vi "setLogMode.vi"(8 "error in (no error)":errorcluster, 10 "LogMode":T1=enum."Logging", 11 "Instrument.Lockin in":refnum<class "Instrument.Lockin.lvclass">) -> (0 "error out":errorcluster, 3 "Instrument.Lockin out":refnum<class "Instrument.Lockin.lvclass">)   [LabVIEW 2019, in "Instrument.Lockin.lvlib" / "Instrument.Lockin.lvclass"]
doc: "Set the state {start, stop, reset, start sweep, stop sweep}"
uses:
  Instrument.Lockin.lvclass
  Typedefs/LogMode--Enum.ctl
  Typedefs/API/Lockin.Commands--Enum.ctl
  Typedefs/API/Lockin.setLogMode--cluster.ctl
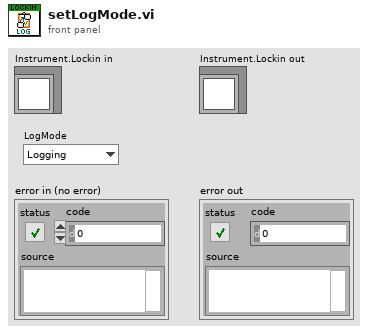
[diagram p1: front panel]
types:
  T1 = typedef "Instrument.Lockin.lvlib/Instrument.Lockin.lvclass/LogMode--Enum.ctl" = enum16{"Heartbeat", "Logging"}
  T2 = typedef "Instrument.Lockin.lvlib/Instrument.Lockin.lvclass/Lockin.setLogMode--cluster.ctl" = cluster{"LogMode":T1}
  T3 = typedef "Instrument.Lockin.lvlib/Instrument.Lockin.lvclass/Lockin.Commands--Enum.ctl" = enum16{"setAO", "setAO_Amplitude", "setAO_DC", "setAO_Frequency", "setAO_Phase", "setAO_Function", "setREF", "setREF_Frequency", "setREF_Phase", "setREF_TC", "setREF_Roll-Off", "setDAQ", "setSampling", "setState", "getState", "getAO", "getAI", "getResults", "getSampling", "getAOconfig", "getREFconfig", "setInputGain", "setOutputGain", "getInputGain", "getOutputGain", "setSamplingFsMode", "getSamplingFsMode", "setSweep", "setSweep_Time", "setSweep_Table", "getStatus", "getSweepResults", "getSweepWaveforms", "setLogMode"}
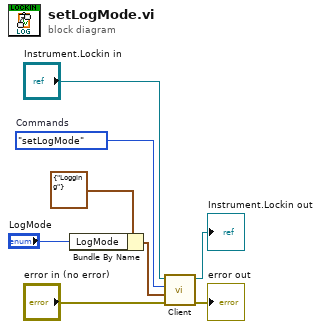
[diagram p0: block diagram]
diagram:
  w6 = Lockin.Commands--Enum."setLogMode"  # Commands
  n1 = Bundle By Name(cluster=T2 {"LogMode"=enum."Logging"} ("setLogging"), "LogMode"="LogMode") -> (w7:T2)
  n2 = call-dynamic "Client.vi"("error in (no error)"="error in (no error)", "Data in"=w7, "Command in"=w6, "Instrument in"="Instrument.Lockin in") -> ("error out"=→"error out":errorcluster, "Instrument out"=→"Instrument.Lockin out":refnum<class "Instrument.Lockin.lvclass">)  [unwired: 4 in, 2 out]
